vi "Fuzzify.vi"(2 "input-value":dbl format="%.2f", 3 "input-name":string, 4 "Controller":T1={"Parameters"={"antecedance"=[{"ling.var."="in1", "x-min"=-1.0, "x-max"=1.0, "setarray"=[{"linguistic term"="NE1", "color"=16711680, "points"=[-1.0, -1.0, -1.0, -2.2351741790771484e-05]}, {"linguistic term"="ZE1", "color"=255, "points"=[-1.0, 0.0, 0.0, 1.0]}, {"linguistic term"="PO1", "color"=26214, "points"=[0.0, 1.0, 1.0, 1.0]}]}, {"ling.var."="in2", "x-min"=-1.0, "x-max"=1.0, "setarray"=[{"linguistic term"="NE2", "color"=16711680, "points"=[-1.0, -1.0, -1.0, 0.0]}, {"linguistic term"="ZE2", "color"=255, "points"=[-1.0, 0.0, 0.0, 1.0]}, {"linguistic term"="PO2", "color"=26214, "points"=[0.0, 1.0, 1.0, 1.0]}]}], "consequence"=[{"ling.var."="out", "x-min"=-1.0, "x-max"=1.0, "setarray"=[{"linguistic term"="NEo", "color"=16711680, "points"=[-1.0, -1.0, -1.0, 0.0]}, {"linguistic term"="ZEo", "color"=255, "points"=[-1.0, 0.0, 0.0, 1.0]}, {"linguistic term"="POo", "color"=26214, "points"=[0.0, 1.0, 1.0, 1.0]}]}], "conclusions"=[3, 3, 3, 3, 3, 3, 3], "degree-of-support"=[1.0, 1.0, 1.0, 1.0, 1.0, 1.0, 1.0], "defu"=[{"inference"=0, "defumethod"=0, "modification"=TRUE, "precision"=0, "no consequence"=0, "defaultvalue"=0.0}]}, "Description"={"Info"={"Path"=path "/HD 1000/Desktop Folder/fuzzylab today/loadsave.vi", "Controller Name"="", "Date"="", "Time"=""}, "Author"="", "Text"=""}} {"Parameters"."defu"."defaultvalue" format="%.2f"; "Parameters"."degree-of-support" step=0.009999999776482582 format="%.2f"; "Parameters"."consequence"."x-min" step=0.009999999776482582 format="%.2f"; "Parameters"."consequence"."x-max" step=0.009999999776482582 format="%.2f"; "Parameters"."consequence"."setarray"."points" step=0.009999999776482582 format="%.2f"; "Parameters"."antecedance"."x-min" step=0.009999999776482582 format="%.2f"; "Parameters"."antecedance"."x-max" step=0.009999999776482582 format="%.2f"; "Parameters"."antecedance"."setarray"."points" step=0.009999999776482582 format="%.2f"}) -> (0 "error out":errorcluster={"status"=FALSE, "code"=0, "source"="no error"}, 1 "fuzzified antecedance":T2 {"fulfillment" format="%.2f"})   [LabVIEW 2017, in "NI_fuzzy logic.lvlib"]
doc: "This VI fuzzifies the precise input value of the linguistic variable specified by the \"name in\" input. For each linguistic term of the linguistic variable the VI supplies the degree of truth of which the term represents the input value. \nIf \"name in\" is left unwired, the controller input is disabled."
uses:
  <vilib>/addons/control/fuzzy/NI_fuzzy logic.lvlib
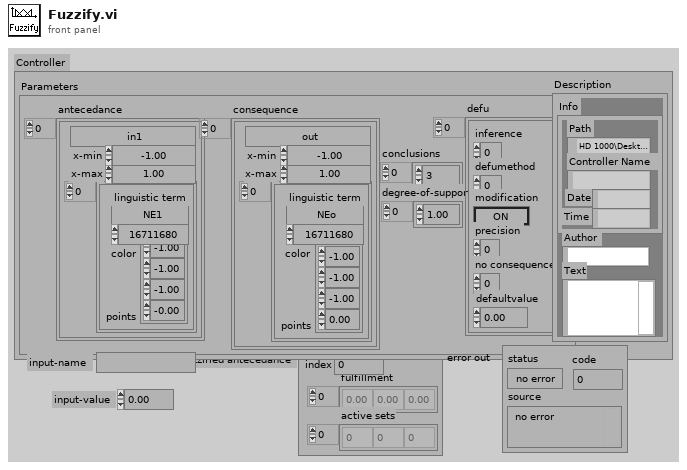
[diagram p1: front panel]
types:
  T1 = cluster{"Parameters":cluster{"antecedance":cluster{"ling.var.":string, "x-min":dbl, "x-max":dbl, "setarray":cluster{"linguistic term":string, "color":u32, "points":dbl[]}[]}[], "consequence":cluster{"ling.var.":string, "x-min":dbl, "x-max":dbl, "setarray":cluster{"linguistic term":string, "color":u32, "points":dbl[]}[]}[], "conclusions":u16[], "degree-of-support":dbl[], "defu":cluster{"inference":u16, "defumethod":u16, "modification":bool, "precision":u16, "no consequence":u16, "defaultvalue":dbl}[]}, "Description":cluster{"Info":cluster{"Path":path, "Controller Name":string, "Date":string, "Time":string}, "Author":string, "Text":string}}
  T2 = cluster{"index":i32, "fulfillment":dbl[], "active sets":i32[]}
  T3 = cluster{"ling.var.":string, "x-min":dbl, "x-max":dbl, "setarray":cluster{"linguistic term":string, "color":u32, "points":dbl[]}[]}[]
  T4 = cluster{"ling.var.":string, "x-min":dbl, "x-max":dbl, "setarray":cluster{"linguistic term":string, "color":u32, "points":dbl[]}[]}
  T5 = cluster{"linguistic term":string, "color":u32, "points":dbl[]}[]
  T6 = cluster{"points[0]":dbl, "points[1]":dbl, "points[2]":dbl, "points[3]":dbl}
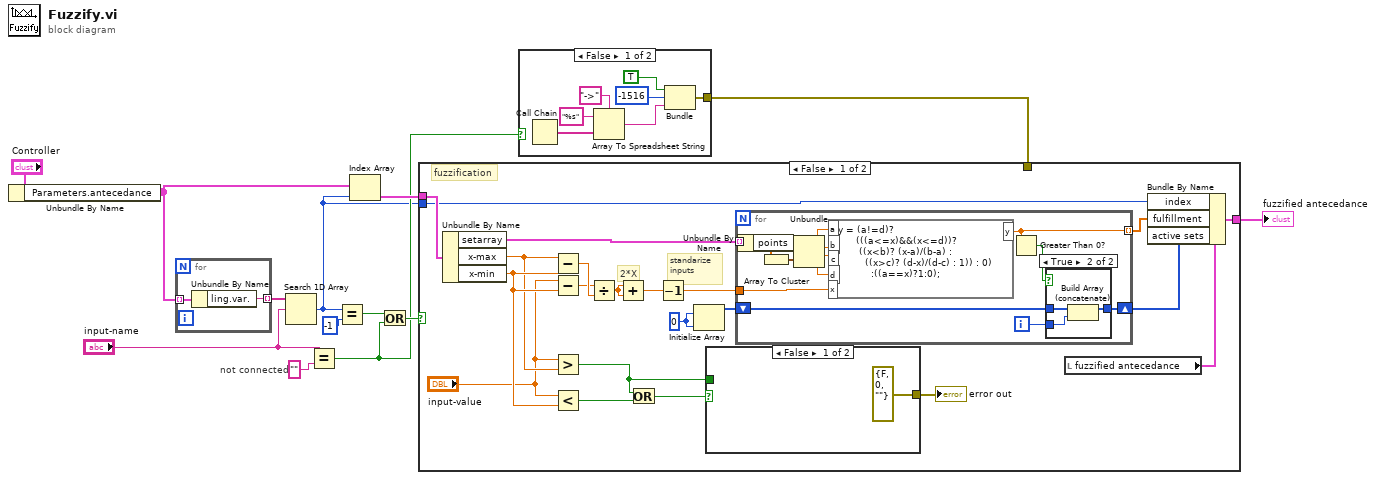
[diagram p0: block diagram]
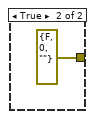
[diagram p2: hidden frame]
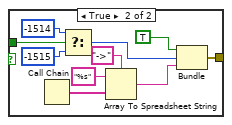
[diagram p3: hidden frame]
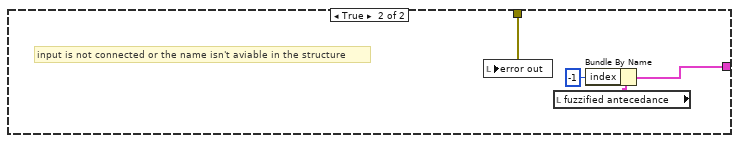
[diagram p5: hidden frame]
diagram:
  # "not connected"
  n1 = Unbundle By Name("Controller") -> ("Parameters.antecedance"=w1:T3)
  n2 = for {
    tunnel: w1 -> [w15] mode=indexing
    tunnel: [w14] -> w8 mode=indexing
    n3 = Unbundle By Name(w15) -> ("ling.var."=w14:string)
  }
  n4 = Search 1D Array(1D array=w8, element="input-name") -> (index of element=w2:i32)  [unwired: 1 out]
  n5 = Equal?(x="input-name", y="") -> (x = y?=w4:bool)
  n6 = Equal?(x=w2, y=-1) -> (x = y?=w10:bool)
  n7 = Index Array(array=w1, index=w2) -> (element=w12:T4)
  n8 = Or(x=w10, y=w4) -> (x .or. y?=w9:bool)
  n9 = case shown="False" w4 {
    tunnel: [w22 cluster{bool, i32, "spreadsheet string":string} {FALSE, 0, "spreadsheet string"=""}] -> w3
    frame False {
      n10 = Call Chain() -> (call chain=w19:string[])
      n11 = Array To Spreadsheet String(delimiter (Tab)="->", array=w19, 3:"%s" ("format string")) -> (spreadsheet string=w16:string)
      n12 = Bundle(TRUE, -1516, "spreadsheet string"=w16) -> (w22:cluster{bool, i32, "spreadsheet string":string})  [unwired: 1 out]
    }
    frame True {
    }
  }
  n13 = case shown="False" w9 {
    tunnel: w12 -> [w36 _]
    tunnel: w3 -> [_ w76]
    tunnel: w2 -> [w29 _]
    tunnel: [w31 w75] -> w5
    frame False {
      w34 = 0
      # "2*X"
      # "fuzzification"
      # "standarize\ninputs"
      n14 = Unbundle By Name(w36) -> ("setarray"=w41:T5, "x-max"=w43:dbl, "x-min"=w44:dbl)
      n15 = Subtract(x=w43, y=w44) -> (x-y=w42:dbl)
      n16 = Subtract(x="input-value", y=w44) -> (x-y=w38:dbl)
      n17 = Greater?(x="input-value", y=w43) -> (0:w27:bool)
      n18 = Less?(x="input-value", y=w44) -> (x < y?=w28:bool)
      n19 = Divide(x=w38, y=w42) -> (x/y=w24:dbl)
      n20 = Add(x=w24, y=w24) -> (x+y=w39:dbl)
      n21 = Or(x=w27, y=w28) -> (x .or. y?=w26:bool)
      n22 = Decrement(x=w39) -> (x-1=w40:dbl)
      n23 = Initialize Array(w34, w34) -> (w33:i32[])
      n24 = case shown="False" w26 {
        tunnel: [cluster{bool, i32, "spreadsheet string":string} {FALSE, 0, "spreadsheet string"=""} w55] -> w25
        tunnel: w27 -> [_ w46]
        frame False {
        }
        frame True {
          n25 = Call Chain() -> (call chain=w53:string[])
          n26 = Select(t=-1514, s=w46, f=-1515) -> (s? t:f=w47:i32)
          n27 = Array To Spreadsheet String(delimiter (Tab)="->", array=w53, 3:"%s" ("format string")) -> (spreadsheet string=w50:string)
          n28 = Bundle(TRUE, w47, "spreadsheet string"=w50) -> (w55:cluster{bool, i32, "spreadsheet string":string})  [unwired: 1 out]
        }
      }
      "error out" <- w25
      n29 = for {
        tunnel: w41 -> [w68] mode=indexing
        tunnel: w40 -> [w66]
        tunnel: [w60] -> w35 mode=indexing
        shift-right: [w58] -> w32
        shift-left: w33 -> [w56]
        i -> [w57]
        # "fuzzify"
        n30 = Unbundle By Name(w68) -> ("points"=w67:dbl[])
        n31 = Array To Cluster(array=w67) -> (cluster=w62:T6)
        n32 = Unbundle(w62) -> ("points[0]"=w65:dbl, "points[1]"=w64:dbl, "points[2]"=w63:dbl, "points[3]"=w61:dbl)
        n33 = formula code="y = (a!=d)?\n      (((a<=x)&&(x<=d))? \n       ((x<b)? (x-a)/(b-a) : \n         ((x>c)? (d-x)/(d-c) : 1)) : 0)\n           :((a==x)?1:0);"("a"=w65, "b"=w64, "c"=w63, "d"=w61, "x"=w66) -> ("y"=w60:dbl)
        n34 = Greater Than 0?(x=w60) -> (x > 0?=w59:bool)
        n35 = case shown="True" w59 {
          tunnel: [w69 w72] -> w58
          tunnel: w57 -> [_ w70]
          tunnel: w56 -> [w69 w71]
          frame False {
          }
          frame True {
            n36 = Build Array (concatenate)(w71, w70) -> (w72:i32[])
          }
        }
      }
      n37 = local read "fuzzified antecedance"() -> (w30:T2)
      n38 = Bundle By Name(cluster=w30, "index"=w29, "fulfillment"=w35, "active sets"=w32) -> (w31:T2)
    }
    frame True {
      # "input is not connected or the name isn't aviable in the structure"
      n39 = local write "error out"(w76) -> ()
      n40 = local read "fuzzified antecedance"() -> (w74:T2)
      n41 = Bundle By Name(cluster=w74, "index"=-1) -> (w75:T2)
    }
  }
  "fuzzified antecedance" <- w5
